vi "Update Tab Page Caption.vi"(8 "error in":errorcluster, 10 "Caption":string[](array[string]), 11 "Pages ref":refnum<vi>[](array[refnum])) -> (0 "error out":errorcluster, 3 "Page ref dup":refnum<vi>[](array[refnum]))   [LabVIEW 2014]
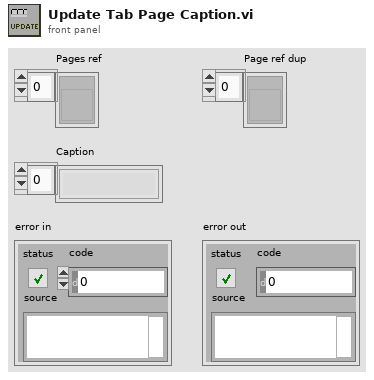
[diagram p1: front panel]
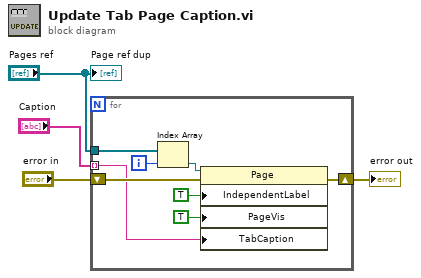
[diagram p0: block diagram]
diagram:
  n1 = for {
    tunnel: "Pages ref" -> [w10]
    shift-right: [w11] -> w3
    shift-left: "error in" -> [w12]
    tunnel: "Caption" -> [w5] mode=indexing
    i -> [w9]
    n2 = Index Array(array=w10, index=w9) -> (element=w8:refnum<vi>)
    n3 = property class="Page"(reference=w8, error in=w12, "IndependentLabel"=TRUE ("Page Visible"), "PageVis"=TRUE ("Independent Label"), "TabCaption"=w5) -> (error out=w11:errorcluster)  [unwired: 1 out]
  }
  "error out" <- w3
  "Page ref dup" <- "Pages ref"
